vi "DeviceNameTCPWriteWithStateMachine.vi"(8 "error in (no error)":errorcluster, 9 "Device name":string, 10 "last scanstart udp":T1, 11 "TCP Network Connection in":refnum<k5>) -> (0 "error out":errorcluster, 3 "TCP Network Connection out":refnum<k5>)   [LabVIEW 2020]
uses:
  Device Drivers/shared/UDP_FGV.ctl
  Device Drivers/UDPComm/UDP FGV control.ctl
  Device Drivers/UDPComm/UDPComm.lvlib
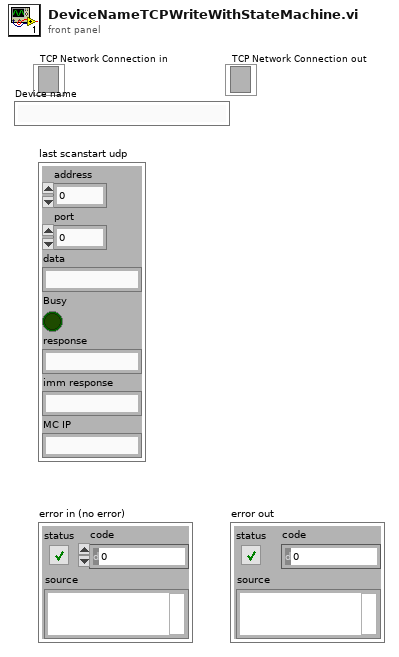
[diagram p1: front panel]
types:
  T1 = typedef "UDP_FGV.ctl" = cluster{"address":u32, "port":u16, "data":string, "Busy":bool, "response":string, "imm response":string, "MC IP":string}
  T2 = typedef "UDP FGV control.ctl" = enum16{"Clear", "WriteToSM", "ReadFromSM", "WriteToUDP", "ReadFromUDP", "LockIP", "UnLockIP"}
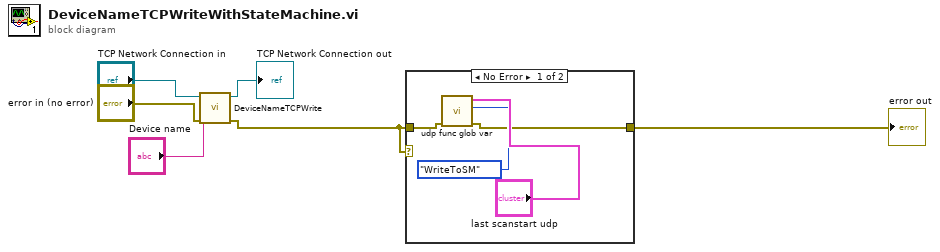
[diagram p0: block diagram]
diagram:
  n1 = call "DeviceNameTCPWrite.vi"("error in (no error)"="error in (no error)", "Device name"="Device name", "connection ID"="TCP Network Connection in") -> ("error out"=w2:errorcluster, "connection ID out"=→"TCP Network Connection out":refnum<k5>)  [unwired: 7 in]
  n2 = case shown="No Error" w2 {
    tunnel: w2 -> [w8 w11]
    tunnel: [w7 w11] -> w3
    frame No Error {
      n3 = call "udp func glob var.vi"("error in"=w8, "Function"=UDP_FGV_control."WriteToSM", "Msg in"="last scanstart udp") -> ("error out"=w7:errorcluster)  [unwired: 6 in, 2 out]
    }
    frame Error {
    }
  }
  "error out" <- w3
